vi "create.vi"(8 "error in":errorcluster, 10 "asset":string, 11 "Nominal Client":refnum<class "Nominal Client.lvclass">) -> (0 "error out":errorcluster, 3 "asset":refnum<class "asset.lvclass">)   [LabVIEW 2020, in "asset.lvclass"]
uses:
  asset.lvclass
  Nominal Client/Nominal Client.lvclass
  asset.lvclass/asset.ctl
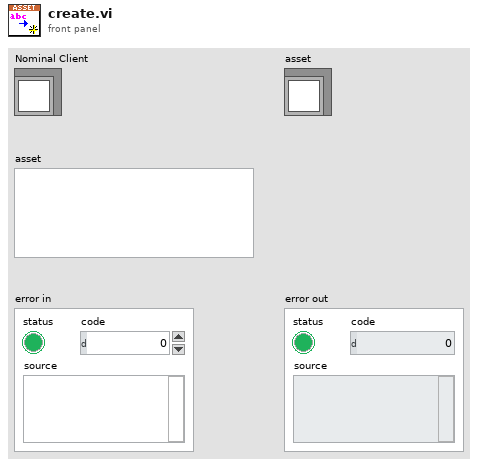
[diagram p1: front panel]
types:
  T1 = typedef "dataScopes.lvlib/links.ctl" = cluster{"URL":string, "Title":string}[]
  T2 = typedef "dataScopes.lvlib/data_scopes.ctl" = T3[]
  T3 = typedef "dataScopes.lvlib/data_scope.ctl" = cluster{"dataScopeName":string, "dataSource":T4, "seriesTags":map{string, string}, "offset":T6}
  T4 = typedef "dataScopes.lvlib/data_source.ctl" = cluster{"type":T5, "rid":string}
  T5 = typedef "dataScopes.lvlib/type.ctl" = enum16{"dataset", "connection", "logSet", "video"}
  T6 = typedef "dataScopes.lvlib/offset.ctl" = cluster{"seconds":i32, "nanos":i32, "picos":i32}
  T7 = cluster{"rid":string, "title":string, "properties":refnum<class "properties.lvclass">, "labels":refnum<class "labels.lvclass">, "Links":T1, "datascopes":T2, "createdAt":timestamp, "updatedAt":timestamp, "attachments":refnum<class "labels.lvclass">, "isStaged":bool, "isArchived":bool, "description":string, "createdBy":string, "type":string}
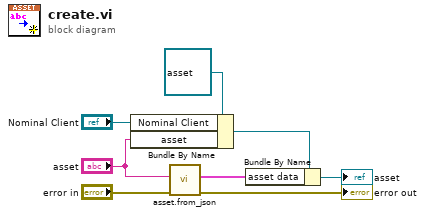
[diagram p0: block diagram]
diagram:
  n1 = Bundle By Name(cluster=refnum<class "asset.lvclass"> refnum ("asset"), "Nominal Client"="Nominal Client", "asset"="asset") -> (w6:refnum<class "asset.lvclass">)
  n2 = call "asset.from_json.vi"("error in"="error in", "asset"="asset") -> ("error out"=→"error out":errorcluster, "Asset Data"=w3:T7)  [unwired: 8 in]
  n3 = Bundle By Name(cluster=w6, "asset data"=w3) -> (→"asset":refnum<class "asset.lvclass">)
